vi "encodeBoolean.vi"(8 "error in (no error)":errorcluster, 10 "Variant":variant) -> (0 "error out":errorcluster, 2 "Array":u8[](array[numeric]) format="%.0x")   [LabVIEW 2016, in "MsgPack.lvlib"]
uses:
  MsgPack.lvlib
  <vilib>/Utility/Data Type/NI_Data Type.lvlib
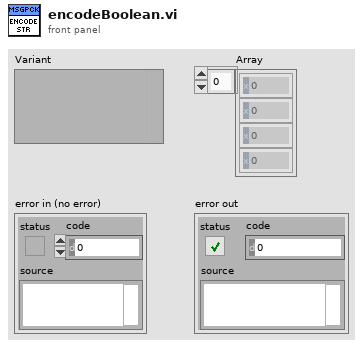
[diagram p1: front panel]
types:
  T1 = typedef "NI_Data Type.lvlib/Data Type.ctl" = enum8{"Invalid Type", "Void", "I8", "I16", "I32", "I64", "U8", "U16", "U32", "U64", "Single Float", "Double Float", "Extended Float", "Single Complex", "Double Complex", "Extended Complex", "Enum U8", "Enum U16", "Enum U32", "Enum U64", "Single Float With Unit", "Double Float With Unit", "Extended Float With Unit", "Single Complex with Unit", "Double Complex with Unit", "Extended Complex with Unit", "Boolean", "String", "Path", "Picture", "Tag", "Array", "Cluster", "Variant", "LV Variant", "Waveform", "Timestamp", "Digital Waveform", "Digital Data", "ExpressData", "Refnum", "External Data", "VI", "Poly VI", "LabVIEW Class Instance", "Fixed Point"}
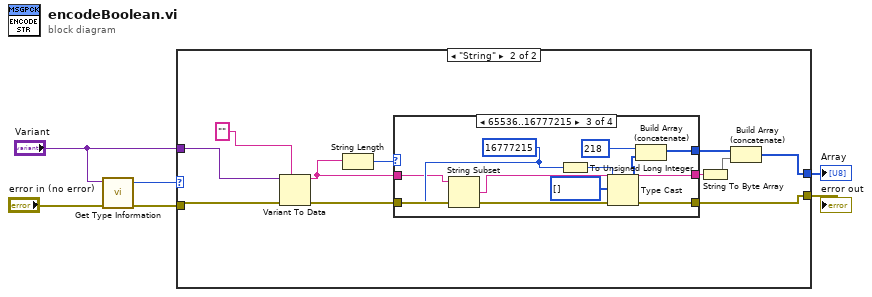
[diagram p0: block diagram]
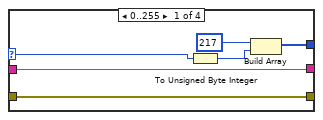
[diagram p3: hidden frame]
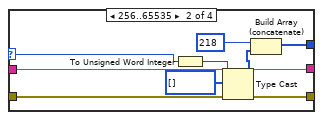
[diagram p4: hidden frame]
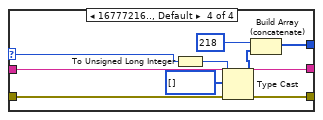
[diagram p5: hidden frame]
diagram:
  n1 = call <vilib>:"Get Type Information.vi"("error in (no error)"="error in (no error)", "Variant"="Variant") -> ("error out"=w5:errorcluster, "Type"=w6:T1)  [unwired: 5 in, 3 out]
  n2 = case shown="\"String\"" w6 {
    tunnel: w5 -> [w7 w18]
    tunnel: "Variant" -> [_ w17]
    tunnel: [_ w9] -> w3
    tunnel: [w7 w8] -> w2
    frame "Invalid Type", Default {
    }
    frame "String" {
      n3 = Variant To Data(error in=w18, type="", Variant=w17) -> (data=w13:string, error out=w14:errorcluster)
      n4 = String Length(string=w13) -> (length=w15:i32)
      n5 = case shown="65536..16777215" w15 {
        selector: w15 -> [w20 w28 _ w45]
        tunnel: w14 -> [w24 w32 w41 w49]
        tunnel: [w24 w32 w41 w49] -> w8
        tunnel: [w22 w30 w33 w47] -> w10
        tunnel: w13 -> [w22 w30 w34 w47]
        tunnel: [w21 w29 w39 w46] -> w12
        frame 0..255 {
          n6 = To Unsigned Byte Integer(number=w20) -> (unsigned 8bit integer=w19:u8)
          n7 = Build Array(u8 217, w19) -> (w21:u8[])
        }
        frame 256..65535 {
          n8 = To Unsigned Word Integer(number=w28) -> (unsigned 16bit integer=w27:u16)
          n9 = Type Cast(type=u8[] [] ("appended array"), x=w27) -> (*(type *) &x=w25:u8[])
          n10 = Build Array (concatenate)(u8 218, w25) -> (w29:u8[])
        }
        frame 65536..16777215 {
          w35 = u32 16777215 ("number")
          n11 = String Subset(string=w34, length (rest)=w35) -> (substring=w33:string)  [unwired: 1 in]
          n12 = To Unsigned Long Integer(number=w35) -> (unsigned 32bit integer=w38:u32)
          n13 = Type Cast(type=u8[] [] ("appended array"), x=w38) -> (*(type *) &x=w36:u8[])
          n14 = Build Array (concatenate)(u8 218, w36) -> (w39:u8[])
        }
        frame 16777216.., Default {
          n15 = To Unsigned Long Integer(number=w45) -> (unsigned 32bit integer=w44:u32)
          n16 = Type Cast(type=u8[] [] ("appended array"), x=w44) -> (*(type *) &x=w42:u8[])
          n17 = Build Array (concatenate)(u8 218, w42) -> (w46:u8[])
        }
      }
      n18 = String To Byte Array(string=w10) -> (unsigned byte array=w11:u8[])
      n19 = Build Array (concatenate)(w12, w11) -> (w9:u8[])
    }
  }
  "Array" <- w3
  "error out" <- w2
